vi "gun_turret_prediction.vi"(8 "delta_t":i64, 9 "Velocity":cluster{"Left":dbl, "Right":dbl}, 10 "Turret":cluster{"R":dbl, "theta":dbl}, 11 "Gun Const":T1) -> (2 "Turret Out":cluster{"R":dbl, "theta":dbl}, 3 "Velocity Lead":cluster{"R":dbl, "theta":dbl})   [LabVIEW 2011]
uses:
  gun_const_t.ctl
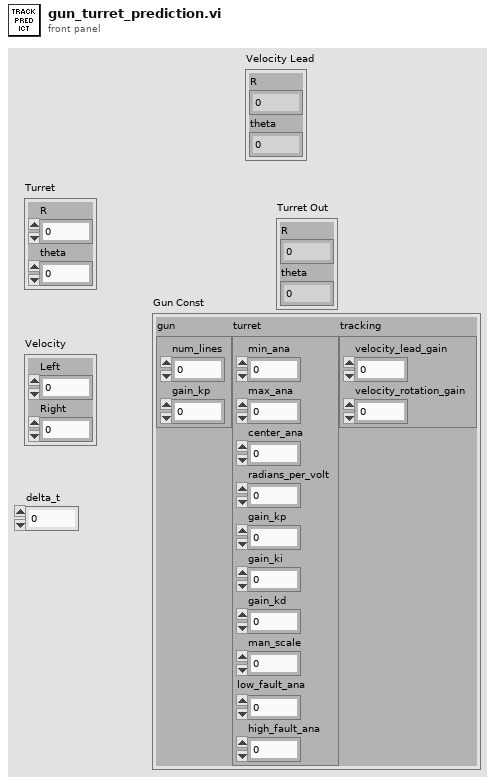
[diagram p1: front panel]
types:
  T1 = typedef "gun_const_t.ctl" = cluster{"gun":cluster{"num_lines":dbl, "gain_kp":dbl}, "turret":cluster{"min_ana":dbl, "max_ana":dbl, "center_ana":dbl, "radians_per_volt":dbl, "gain_kp":dbl, "gain_ki":dbl, "gain_kd":dbl, "man_scale":dbl, "low_fault_ana":dbl, "high_fault_ana":dbl}, "tracking":cluster{"velocity_lead_gain":dbl, "velocity_rotation_gain":dbl}}
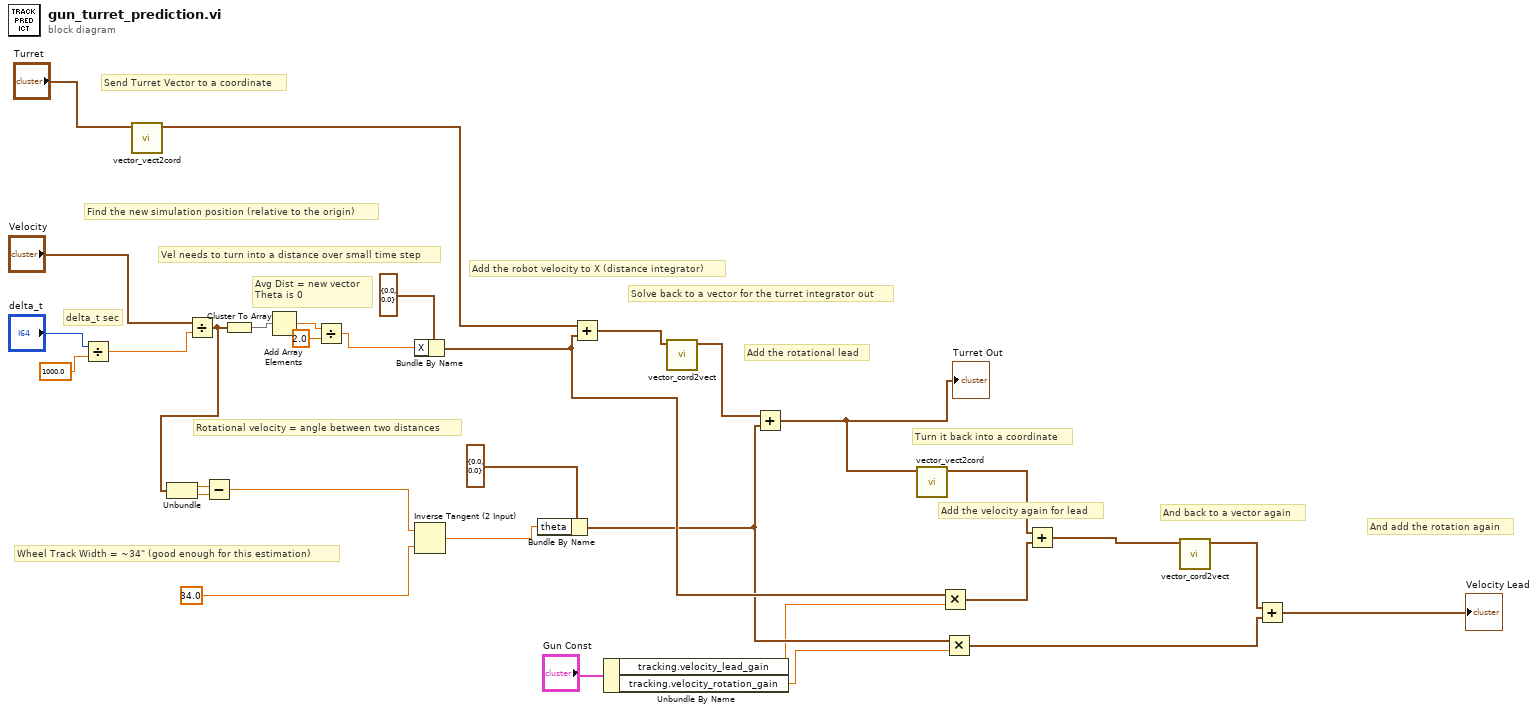
[diagram p0: block diagram]
diagram:
  # "And add the rotation again"
  # "And back to a vector again"
  # "Add the velocity again for lead"
  # "Turn it back into a coordinate"
  # "Add the rotational lead"
  # "Solve back to a vector for the turret integrator out"
  # "Add the robot velocity to X (distance integrator)"
  # "Wheel Track Width = ~34\" (good enough for this estimation)"
  # "Rotational velocity = angle between two distances"
  # "Avg Dist = new vector\nTheta is 0"
  # "Vel needs to turn into a distance over small time step"
  # "delta_t sec"
  # "Find the new simulation position (relative to the origin)"
  # "Send Turret Vector to a coordinate"
  n1 = Divide(x="delta_t", y=1000.0) -> (x/y=w28:dbl)
  n2 = call "vector_vect2cord.vi"("Vector"="Turret") -> ("Coordinate"=w17:cluster{"X":dbl, "Y":dbl})  [unwired: 10 in]
  n3 = Divide(x="Velocity", y=w28) -> (x/y=w22:cluster{"Left":dbl, "Right":dbl})
  n4 = Unbundle(w22) -> ("Left"=w24:dbl, "Right"=w23:dbl)
  n5 = Subtract(x=w24, y=w23) -> (x-y=w20:dbl)
  n6 = Cluster To Array(cluster=w22) -> (array=w27:dbl[])
  n7 = Add Array Elements(numeric array=w27) -> (sum=w26:dbl)
  n8 = Divide(x=w26, y=2.0) -> (x/y=w18:dbl)
  n9 = Bundle By Name(cluster=cluster{"X":dbl, "Y":dbl} {"X"=0.0, "Y"=0.0} ("Coordinate"), "X"=w18) -> (w11:cluster{"X":dbl, "Y":dbl})
  n10 = Inverse Tangent (2 Input)(1:34.0, 2:w20) -> (0:w14:dbl)
  n11 = Bundle By Name(cluster=cluster{"R":dbl, "theta":dbl} {"R"=0.0, "theta"=0.0} ("Vector"), "theta"=w14) -> (w7:cluster{"R":dbl, "theta":dbl})
  n12 = Add(x=w17, y=w11) -> (x+y=w16:cluster{"X":dbl, "Y":dbl})
  n13 = Unbundle By Name("Gun Const") -> ("tracking.velocity_lead_gain"=w2:dbl, "tracking.velocity_rotation_gain"=w1:dbl)
  n14 = call "vector_cord2vect.vi"("Coordinate"=w16) -> ("Vector"=w13:cluster{"R":dbl, "theta":dbl})  [unwired: 10 in]
  n15 = Add(x=w13, y=w7) -> (x+y=w12:cluster{"R":dbl, "theta":dbl})
  "Turret Out" <- w12
  n16 = call "vector_vect2cord.vi"("Vector"=w12) -> ("Coordinate"=w10:cluster{"X":dbl, "Y":dbl})  [unwired: 10 in]
  n17 = Multiply(x=w11, y=w2) -> (x*y=w9:cluster{"X":dbl, "Y":dbl})
  n18 = Multiply(x=w7, y=w1) -> (x*y=w5:cluster{"R":dbl, "theta":dbl})
  n19 = Add(x=w10, y=w9) -> (x+y=w8:cluster{"X":dbl, "Y":dbl})
  n20 = call "vector_cord2vect.vi"("Coordinate"=w8) -> ("Vector"=w6:cluster{"R":dbl, "theta":dbl})  [unwired: 10 in]
  n21 = Add(x=w6, y=w5) -> (x+y=→"Velocity Lead":cluster{"R":dbl, "theta":dbl})
